vi "UDPreceveur.vi"() -> ()   [LabVIEW 2019]
uses:
  <vilib>/myRIO/Instrument Drivers/Utilities/Utilities.lvlib
panel:
  out "error out":errorcluster
  in  "Stop":bool
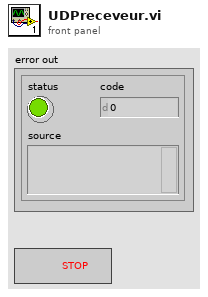
[diagram p1: front panel]
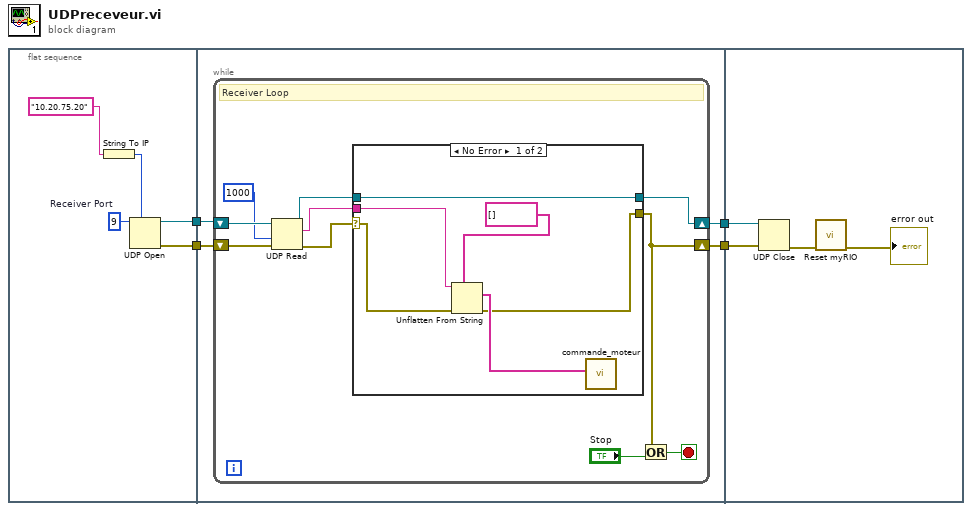
[diagram p0: block diagram]
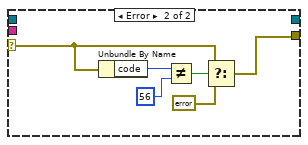
[diagram p2: hidden frame]
diagram:
  n1 = flat-sequence {
    tunnel: [w8] -> w4
    tunnel: [w7] -> w3
    tunnel: [w13] -> w2
    tunnel: [w12] -> w1
    tunnel: w4 -> [w11]
    tunnel: w3 -> [w10]
    tunnel: w2 -> [w38]
    tunnel: w1 -> [w39]
    frame #0 {
      w9 = u16 9  # Receiver Port
      n2 = String To IP(1:"10.20.75.20") -> (0:w5:u32)
      n3 = UDP Open(7:w5, 11:w9) -> (port=w8:refnum<k16>, 0:w7:errorcluster)  [unwired: 3 in, 1 out]
    }
    frame #1 {
      n4 = while {
        shift-right: [w15] -> w12
        shift-left: w10 -> [w19]
        shift-right: [w18] -> w13
        shift-left: w11 -> [w20]
        stop <- w22 stop-if-true
        # "Receiver Loop"
        n5 = UDP Read(connection ID=w20, timeout ms (25000)=1000, 8:w19) -> (data out=w21:string, error out=w14:errorcluster, 3:w17:refnum<k16>)  [unwired: 1 in, 2 out]
        n6 = case shown="No Error" w14 {
          selector: w14 -> [w24 w31]
          tunnel: [w26 w30] -> w15
          tunnel: w21 -> [w27 _]
          tunnel: [w25 _] -> w18
          tunnel: w17 -> [w25 _]
          frame No Error {
            n7 = Unflatten From String(type=string[] [], binary string=w27, error in (no error)=w24) -> (value=w29:string[], error out=w26:errorcluster)  [unwired: 2 in, 1 out]
            n8 = call "commande_moteur.vi"("liste commande"=w29) -> ()  [unwired: 11 in]
          }
          frame Error {
            n9 = Unbundle By Name(w31) -> ("code"=w33:i32)
            n10 = Not Equal?(x=w33, y=56) -> (x != y?=w32:bool)
            n11 = Select(t=w31, s=w32, f=errorcluster {"status"=FALSE, "code"=0, "source"=""} ("error out")) -> (s? t:f=w30:errorcluster)
          }
        }
        n12 = Or(x=w15, y="Stop") -> (x .or. y?=w22:bool)
      }
    }
    frame #2 {
      n13 = UDP Close(connection ID=w38, 8:w39) -> (error out=w37:errorcluster)  [unwired: 1 out]
      n14 = call <vilib>:"Reset myRIO.vi"("error in (no error)"=w37) -> ("error out"=→"error out":errorcluster)  [unwired: 10 in]
    }
  }
